vi "Message.vi"(9 "TorF":bool, 11 "Data In":T1) -> (3 "Data Out":T1)   [LabVIEW 2014]
uses:
  controls/Data1.ctl
panel:
  # "日      期"
  # "機       種"
  # "機       號"
  # "商品條碼"
  # "OK"
  # "台"
  # "NG"
  # "台"
  # "總計"
  # "台"
  # "日      期"
  # "機       種"
  # "機       號"
  # "商品條碼"
  # "OK"
  # "台"
  # "NG"
  # "台"
  # "總計"
  # "台"
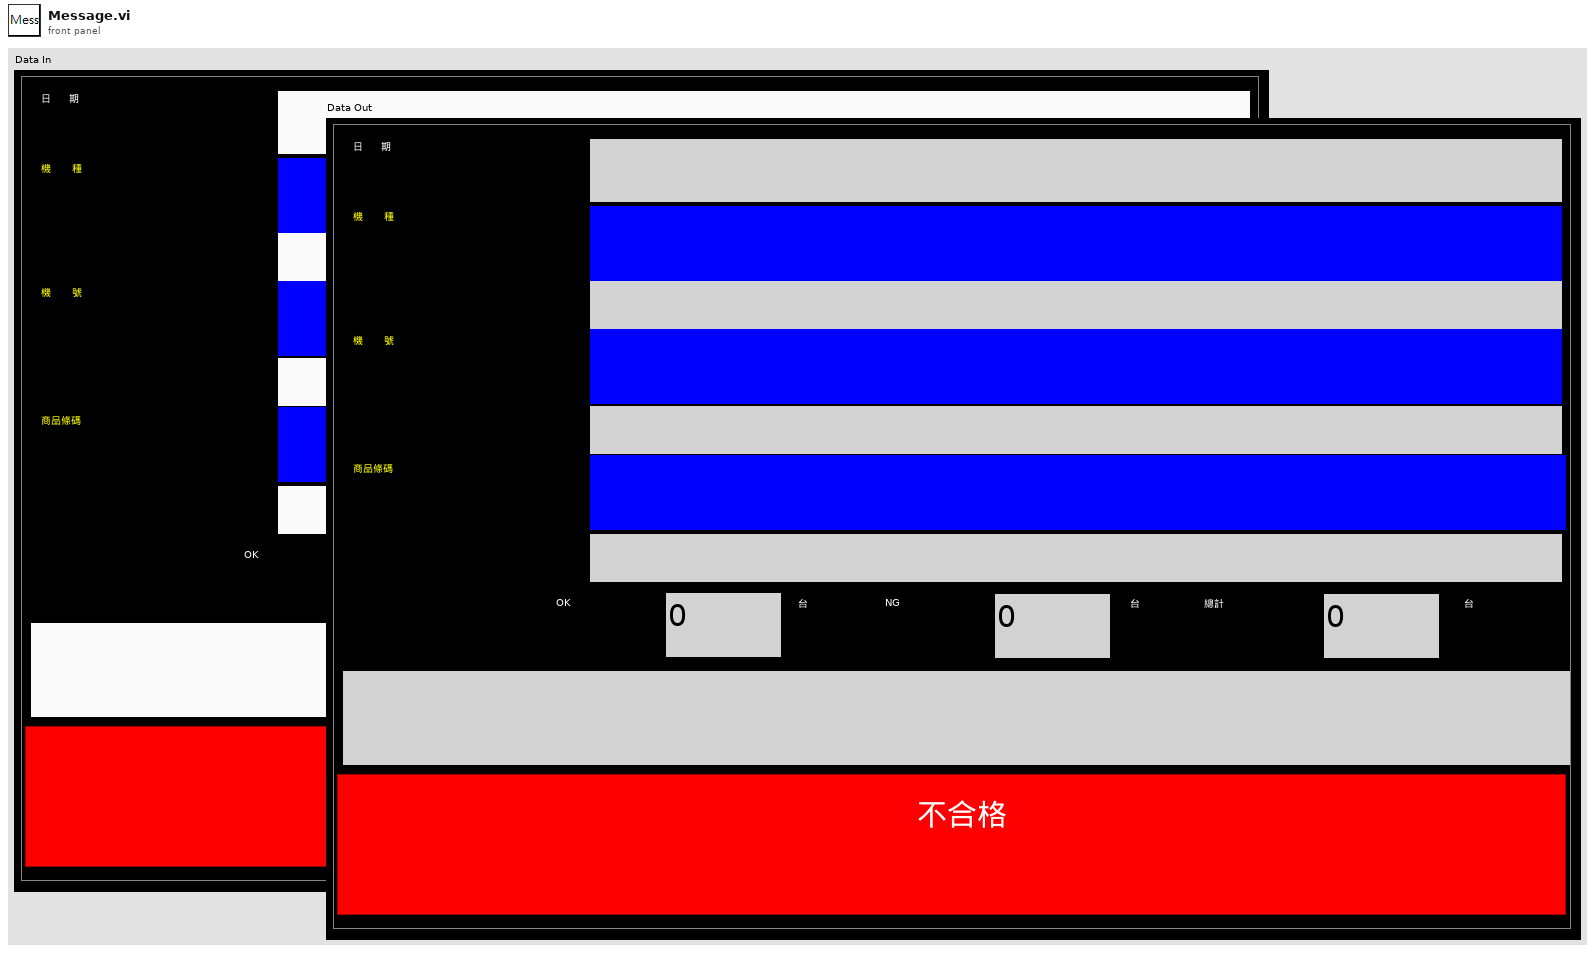
[diagram p1: front panel]
types:
  T1 = typedef "Data1.ctl" = cluster{"Date":string, "BarCode1":string, "BarCode2":string, "BarCode3":string, "Message":string, "OK Count":u16, "NG Count":u16, "Total Count":u16, "ModelData":string[][], "OK&NG":bool, "COM1":refnum<visa-resource-name>, "COM2":refnum<visa-resource-name>, "IO":i32, "Time":u32, "TCP":refnum<k5>, "TCP 2":refnum<k5>, "COM1 2":refnum<visa-resource-name>, "CheckPars":string, "BarCode1_1":string, "BarCode2_1":string, "BarCode3_1":string}
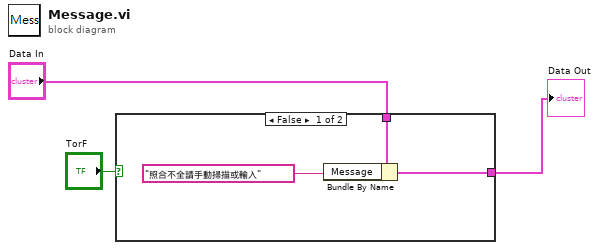
[diagram p0: block diagram]
diagram:
  n1 = case shown="False" "TorF" {
    tunnel: "Data In" -> [w5 w7]
    tunnel: [w4 w7] -> w1
    frame False {
      n2 = Bundle By Name(cluster=w5, "Message"="照合不全請手動掃描或輸入" ("string")) -> (w4:T1)
    }
    frame True {
    }
  }
  "Data Out" <- w1
